vi "pp3_log_toString_trial.vi"(8 "State Info In":T1={"Curr  tr"=0, "Curr (ms)"=0, "Cum (ms)"=0, "Run loop diff"=0, "Tone countdown (ms)"=0, "Countdown (ms)"=0, "Curr State"=enum."0 NULL", "Prev State"=enum."1 Habituation", "Rw"=FALSE, "Sw"=FALSE, "Tone\nGate"=FALSE, "Punish"=FALSE, "Current DAQ DO Int"=0, "Current Loaded Trial"={"Trial Type Number"=1, "Trial Type"=enum."GO", "Trial Weight"=100, "Shock (mA)"=0.3, "Duration (ms)"=0.25, "Sound Type"=enum."04 FM Sweep", "Stim P1"=4000.0, "Stim P2"=0.0, "Stim P3"=0.0, "Stim P4"=2000.0, "DAQ Amplitude (V)"=0.25}, "Next Trial (for display purposes)"={"Trial Type Number"=1, "Trial Type"=enum."GO", "Trial Weight"=100, "Shock (mA)"=0.3, "Duration (ms)"=0.25, "Sound Type"=enum."04 FM Sweep", "Stim P1"=4000.0, "Stim P2"=0.0, "Stim P3"=0.0, "Stim P4"=2000.0, "DAQ Amplitude (V)"=0.25}, "Total trials memo"=0, "State start cum memo (ms)"=0, "Last dur jump time memo (ms)"=0, "Last dur shock time memo (ms)"=0, "Tone repeat memo (ms)"=0, "Webcam on"=FALSE, "Webcam recording"=FALSE, "State update flag"=FALSE, "Last loaded shock voltage"=0.0, "Vid upd"=enum."0"} {"Current DAQ DO Int" format="%016b"; "Next Trial (for display purposes)"."DAQ Amplitude (V)" min=0.0 max=5.0 format="%_6g"; "Next Trial (for display purposes)"."Shock (mA)" min=-1.0 max=5.0; "Next Trial (for display purposes)"."Trial Weight" step=1; "Next Trial (for display purposes)"."Duration (ms)" min=0.0 max=1.0; "Next Trial (for display purposes)"."Trial Type Number" min=1 max=256 step=1; "Current Loaded Trial"."DAQ Amplitude (V)" min=0.0 max=5.0 format="%_6g"; "Current Loaded Trial"."Shock (mA)" min=-1.0 max=5.0; "Current Loaded Trial"."Trial Weight" step=1; "Current Loaded Trial"."Duration (ms)" min=0.0 max=1.0; "Current Loaded Trial"."Trial Type Number" min=1 max=256 step=1}) -> (0 "TRIALMEMO String":string, 3 "spreadsheet string":string)   [LabVIEW 2013]
uses:
  pp3_CTL_StateInfo.ctl
  pp2_CTL_State.ctl
  pp3_CTL_Trial.ctl
  pp3_CTL_TrialType.ctl
  labolabo2/waveforms/WFTypes.ctl
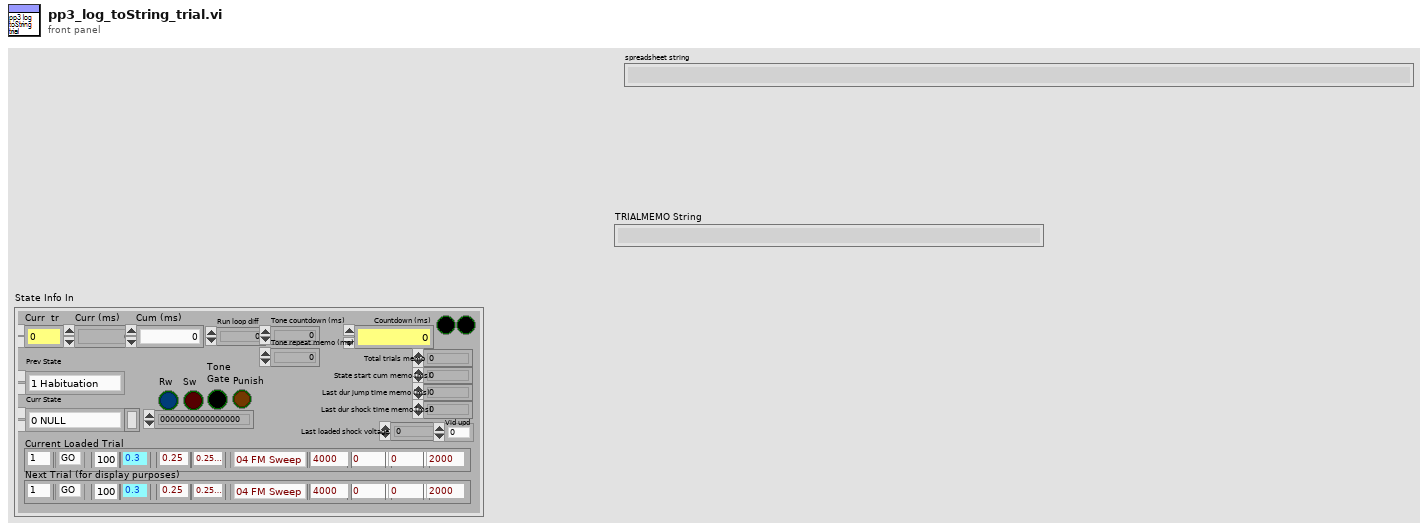
[diagram p1: front panel]
types:
  T1 = typedef "pp3_CTL_StateInfo.ctl" = cluster{"Curr  tr":u16, "Curr (ms)":u32, "Cum (ms)":i64, "Run loop diff":i64, "Tone countdown (ms)":i64, "Countdown (ms)":i64, "Curr State":T2, "Prev State":T2, "Rw":bool, "Sw":bool, "Tone\nGate":bool, "Punish":bool, "Current DAQ DO Int":u16, "Current Loaded Trial":T3, "Next Trial (for display purposes)":T3, "Total trials memo":i64, "State start cum memo (ms)":i64, "Last dur jump time memo (ms)":i64, "Last dur shock time memo (ms)":i64, "Tone repeat memo (ms)":i64, "Webcam on":bool, "Webcam recording":bool, "State update flag":bool, "Last loaded shock voltage":dbl, "Vid upd":enum16{"0", "1", "2", "3", "4", "5", "6", "7", "8", "9"}}
  T2 = typedef "pp2_CTL_State.ctl" = enum8{"0 NULL", "1 Habituation", "2 (Load Trial)", "3 Stay Period", "4 Load Audio/Click Delay", "5 GO Trial", "6 GO Jumped", "7 GO Timeout", "8 NOGO Trial", "9 NOGO Jumped", "10 NOGO Timeout", "11 TEST Trial", "12 TEST Jumped", "13 TEST Timeout", "14 Intertrial Interval", "15 Done"}
  T3 = typedef "pp3_CTL_Trial.ctl" = cluster{"Trial Type Number":i16, "Trial Type":T4, "Trial Weight":u32, "Shock (mA)":dbl, "Duration (ms)":dbl, "Sound Type":T5, "Stim P1":dbl, "Stim P2":dbl, "Stim P3":dbl, "Stim P4":dbl, "DAQ Amplitude (V)":dbl}
  T4 = typedef "pp3_CTL_TrialType.ctl" = enum16{"OFF", "GO", "NOGO", "TEST"}
  T5 = typedef "WFTypes.ctl" = enum16{"00 NULL", "01 DC", "02 Noise", "03 Pure Tone", "04 FM Sweep"}
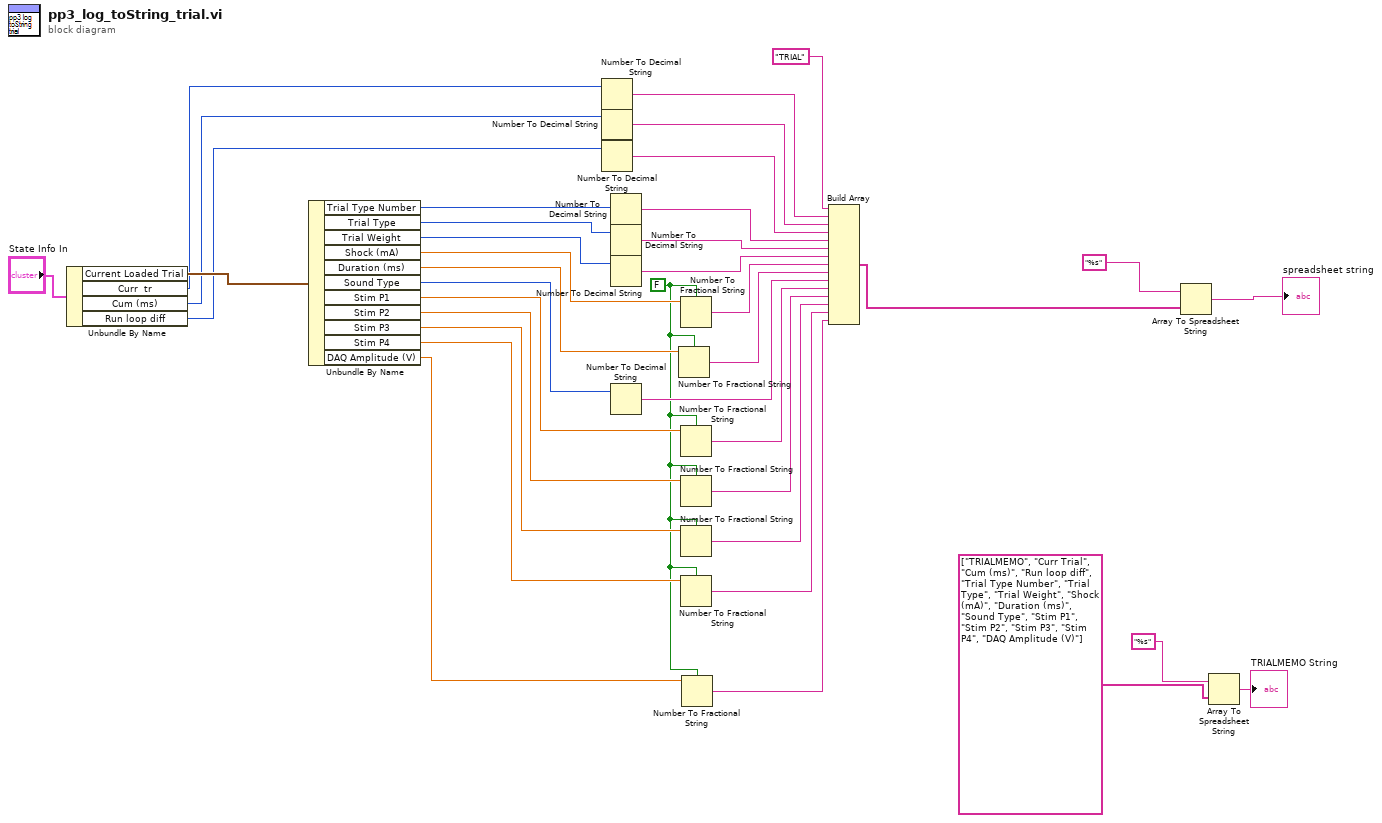
[diagram p0: block diagram]
diagram:
  w3 = FALSE
  n1 = Unbundle By Name("State Info In") -> ("Current Loaded Trial"=w10:T3, "Curr  tr"=w9:u16, "Cum (ms)"=w8:i64, "Run loop diff"=w7:i64)
  n2 = Unbundle By Name(w10) -> ("Trial Type Number"=w33:i16, "Trial Type"=w32:T4, "Trial Weight"=w31:u32, "Shock (mA)"=w22:dbl, "Duration (ms)"=w21:dbl, "Sound Type"=w30:T5, "Stim P1"=w20:dbl, "Stim P2"=w19:dbl, "Stim P3"=w18:dbl, "Stim P4"=w17:dbl, "DAQ Amplitude (V)"=w2:dbl)
  n3 = Number To Decimal String(number=w9) -> (decimal integer string=w6:string)  [unwired: 1 in]
  n4 = Number To Decimal String(number=w8) -> (decimal integer string=w5:string)  [unwired: 1 in]
  n5 = Number To Decimal String(number=w7) -> (decimal integer string=w4:string)  [unwired: 1 in]
  n6 = Number To Decimal String(number=w33) -> (decimal integer string=w34:string)  [unwired: 1 in]
  n7 = Number To Decimal String(number=w32) -> (decimal integer string=w38:string)  [unwired: 1 in]
  n8 = Number To Decimal String(number=w31) -> (decimal integer string=w37:string)  [unwired: 1 in]
  n9 = Number To Decimal String(number=w30) -> (decimal integer string=w27:string)  [unwired: 1 in]
  n10 = Number To Fractional String(use system decimal point (T)=w3, number=w21) -> (F-format string=w28:string)  [unwired: 2 in]
  n11 = Number To Fractional String(use system decimal point (T)=w3, number=w22) -> (F-format string=w29:string)  [unwired: 2 in]
  n12 = Number To Fractional String(use system decimal point (T)=w3, number=w20) -> (F-format string=w26:string)  [unwired: 2 in]
  n13 = Number To Fractional String(use system decimal point (T)=w3, number=w19) -> (F-format string=w25:string)  [unwired: 2 in]
  n14 = Number To Fractional String(use system decimal point (T)=w3, number=w18) -> (F-format string=w24:string)  [unwired: 2 in]
  n15 = Number To Fractional String(use system decimal point (T)=w3, number=w17) -> (F-format string=w23:string)  [unwired: 2 in]
  n16 = Number To Fractional String(use system decimal point (T)=w3, number=w2) -> (F-format string=w1:string)  [unwired: 2 in]
  n17 = Build Array("TRIAL" ("element"), w6, w5, w4, w34, w38, w37, w29, w28, w27, w26, w25, w24, w23, w1) -> (w35:string[])
  n18 = Array To Spreadsheet String(array=w35, 3:"%s" ("format string")) -> (spreadsheet string=→"spreadsheet string":string)  [unwired: 1 in]
  n19 = Array To Spreadsheet String(array=string[] ["TRIALMEMO", "Curr Trial", "Cum (ms)", "Run loop diff", "Trial Type Number", "Trial Type", "Trial Weight", "Shock (mA)", "Duration (ms)", "Sound Type", "Stim P1", "Stim P2", "Stim P3", "Stim P4", "DAQ Amplitude (V)"], 3:"%s" ("format string")) -> (spreadsheet string=→"TRIALMEMO String":string)  [unwired: 1 in]
